vi "战舰移动限制+导弹敌机.vi"() -> ()   [LabVIEW 2018]
panel:
  in  "敌机数量":dbl
  in  "敌机速度":dbl
  out "敌机":picture
  out "按键":dbl
  out "战舰":T1
  out "激光武器1":T2
  out "激光武器 2":T2
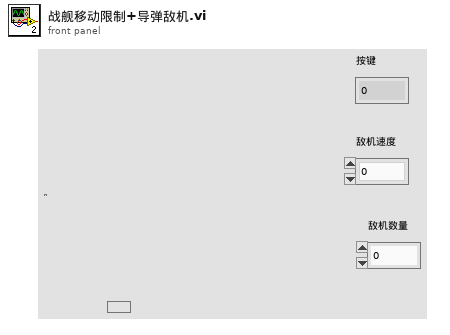
[diagram p1: front panel]
types:
  T1 = typedef "战列巡洋舰.ctl" = picture
  T2 = typedef "战列巡洋舰_激光武器.ctl" = picture
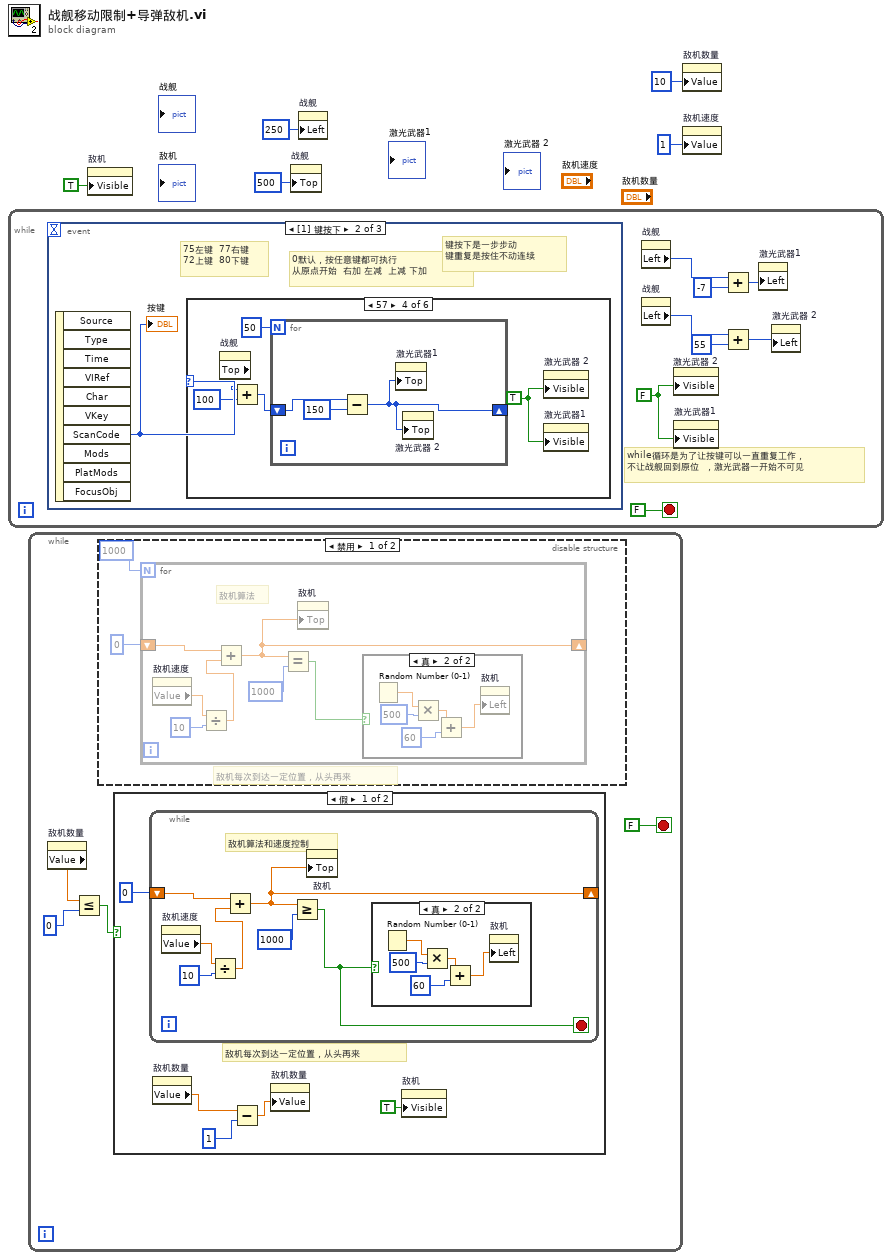
[diagram p0: block diagram]
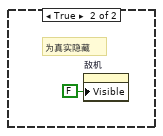
[diagram p3: hidden frame]
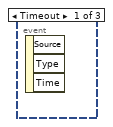
[diagram p6: hidden frame]
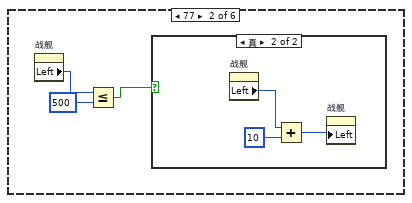
[diagram p8: hidden frame]
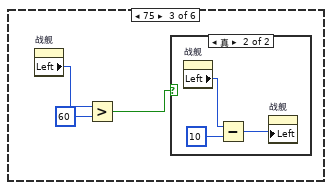
[diagram p10: hidden frame]
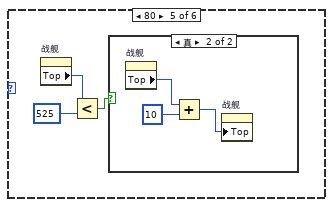
[diagram p12: hidden frame]
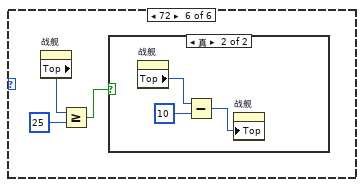
[diagram p14: hidden frame]
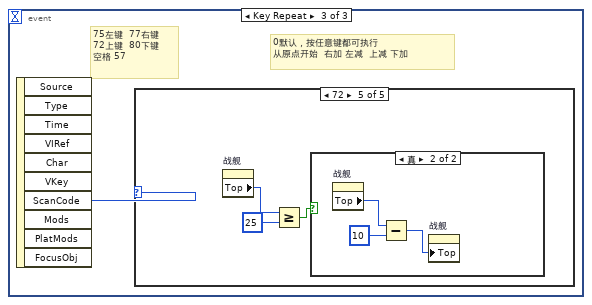
[diagram p16: hidden frame]
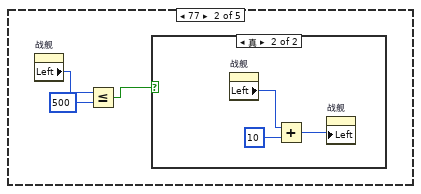
[diagram p18: hidden frame]
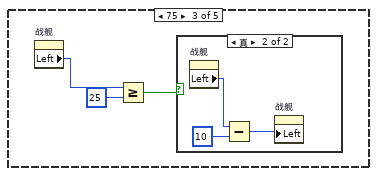
[diagram p20: hidden frame]
diagram:
  n1 = while {
    stop <- FALSE stop-if-true
    w6 = FALSE
    # "while循环是为了让按键可以一直重复工作，\n不让战舰回到原位  ，激光武器一开始不可见"
    n2 = event shown="[1] 键按下" {
      selector: _ -> [_ _ _]
      dyn-events: _ -> [_ _ _]
      timeout: _ -> [_ _ _]
      event Timeout {
        n3 = event-data() -> ()  [unwired: 1 in, 3 out]
      }
      event Key Down {
        # "键按下是一步步动\n键重复是按住不动连续"
        # "75左键  77右键\n72上键  80下键"
        # "0默认，按任意键都可执行\n从原点开始  右加 左减  上减 下加"
        n4 = event-data() -> ("ScanCode"=w14:i16)  [unwired: 1 in, 9 out]
        "按键" <- w14
        n5 = case shown="57" w14 {
          frame 0, Default {
          }
          frame 77 {
            n6 = property on="战舰" class="Pict (严格)"() -> ("Left"=w17:i32)  [unwired: 2 in, 2 out]
            n7 = Less Or Equal?(x=w17, y=500) -> (x <= y?=w15:bool)
            n8 = case shown="真" w15 {
              frame False {
              }
              frame True {
                n9 = property on="战舰" class="Pict (严格)"() -> ("Left"=w19:i32)  [unwired: 2 in, 2 out]
                n10 = Add(x=w19, y=10) -> (x+y=w20:i32)
                n11 = property on="战舰" class="Pict (严格)"("Left"=w20) -> ()  [unwired: 2 in, 2 out]
              }
            }
          }
          frame 75 {
            n12 = property on="战舰" class="Pict (严格)"() -> ("Left"=w23:i32)  [unwired: 2 in, 2 out]
            n13 = Greater?(x=w23, y=60) -> (0:w21:bool)
            n14 = case shown="真" w21 {
              frame False {
              }
              frame True {
                n15 = property on="战舰" class="Pict (严格)"() -> ("Left"=w25:i32)  [unwired: 2 in, 2 out]
                n16 = Subtract(x=w25, y=10) -> (x-y=w26:i32)
                n17 = property on="战舰" class="Pict (严格)"("Left"=w26) -> ()  [unwired: 2 in, 2 out]
              }
            }
          }
          frame 57 {
            w27 = TRUE
            n18 = property on="战舰" class="Pict (严格)"() -> ("Top"=w30:i32)  [unwired: 2 in, 2 out]
            n19 = Add(x=w30, y=100) -> (x+y=w28:i32)
            n20 = for {
              N: 50 -> [_]
              shift-right: [w32] -> _
              shift-left: w28 -> [w34]
              n21 = Subtract(x=w34, y=150) -> (x-y=w32:i32)
              n22 = property on="激光武器1" class="Pict (严格)"("Top"=w32) -> ()  [unwired: 2 in, 2 out]
              n23 = property on="激光武器 2" class="Pict (严格)"("Top"=w32) -> ()  [unwired: 2 in, 2 out]
            }
            n24 = property on="激光武器 2" class="Pict (严格)"("Visible"=w27) -> ()  [unwired: 2 in, 2 out]
            n25 = property on="激光武器1" class="Pict (严格)"("Visible"=w27) -> ()  [unwired: 2 in, 2 out]
          }
          frame 80 {
            n26 = property on="战舰" class="Pict (严格)"() -> ("Top"=w37:i32)  [unwired: 2 in, 2 out]
            n27 = Less?(x=w37, y=525) -> (x < y?=w35:bool)
            n28 = case shown="真" w35 {
              frame False {
              }
              frame True {
                n29 = property on="战舰" class="Pict (严格)"() -> ("Top"=w39:i32)  [unwired: 2 in, 2 out]
                n30 = Add(x=w39, y=10) -> (x+y=w38:i32)
                n31 = property on="战舰" class="Pict (严格)"("Top"=w38) -> ()  [unwired: 2 in, 2 out]
              }
            }
          }
          frame 72 {
            n32 = property on="战舰" class="Pict (严格)"() -> ("Top"=w43:i32)  [unwired: 2 in, 2 out]
            n33 = Greater Or Equal?(x=w43, y=25) -> (x >= y?=w42:bool)
            n34 = case shown="真" w42 {
              frame False {
              }
              frame True {
                n35 = property on="战舰" class="Pict (严格)"() -> ("Top"=w46:i32)  [unwired: 2 in, 2 out]
                n36 = Subtract(x=w46, y=10) -> (x-y=w45:i32)
                n37 = property on="战舰" class="Pict (严格)"("Top"=w45) -> ()  [unwired: 2 in, 2 out]
              }
            }
          }
        }
      }
      event Key Repeat {
        # "75左键  77右键\n72上键  80下键\n空格 57"
        # "0默认，按任意键都可执行\n从原点开始  右加 左减  上减 下加"
        n38 = event-data() -> ("ScanCode"=w47:i16)  [unwired: 1 in, 9 out]
        n39 = case shown="72" w47 {
          frame 0, Default {
          }
          frame 77 {
            n40 = property on="战舰" class="Pict (严格)"() -> ("Left"=w50:i32)  [unwired: 2 in, 2 out]
            n41 = Less Or Equal?(x=w50, y=500) -> (x <= y?=w49:bool)
            n42 = case shown="真" w49 {
              frame False {
              }
              frame True {
                n43 = property on="战舰" class="Pict (严格)"() -> ("Left"=w52:i32)  [unwired: 2 in, 2 out]
                n44 = Add(x=w52, y=10) -> (x+y=w53:i32)
                n45 = property on="战舰" class="Pict (严格)"("Left"=w53) -> ()  [unwired: 2 in, 2 out]
              }
            }
          }
          frame 75 {
            n46 = property on="战舰" class="Pict (严格)"() -> ("Left"=w56:i32)  [unwired: 2 in, 2 out]
            n47 = Greater Or Equal?(x=w56, y=25) -> (x >= y?=w55:bool)
            n48 = case shown="真" w55 {
              frame False {
              }
              frame True {
                n49 = property on="战舰" class="Pict (严格)"() -> ("Left"=w59:i32)  [unwired: 2 in, 2 out]
                n50 = Subtract(x=w59, y=10) -> (x-y=w58:i32)
                n51 = property on="战舰" class="Pict (严格)"("Left"=w58) -> ()  [unwired: 2 in, 2 out]
              }
            }
          }
          frame 80 {
            n52 = property on="战舰" class="Pict (严格)"() -> ("Top"=w62:i32)  [unwired: 2 in, 2 out]
            n53 = Less Or Equal?(x=w62, y=525) -> (x <= y?=w61:bool)
            n54 = case shown="真" w61 {
              frame False {
              }
              frame True {
                n55 = property on="战舰" class="Pict (严格)"() -> ("Top"=w64:i32)  [unwired: 2 in, 2 out]
                n56 = Add(x=w64, y=10) -> (x+y=w63:i32)
                n57 = property on="战舰" class="Pict (严格)"("Top"=w63) -> ()  [unwired: 2 in, 2 out]
              }
            }
          }
          frame 72 {
            n58 = property on="战舰" class="Pict (严格)"() -> ("Top"=w68:i32)  [unwired: 2 in, 2 out]
            n59 = Greater Or Equal?(x=w68, y=25) -> (x >= y?=w67:bool)
            n60 = case shown="真" w67 {
              frame False {
              }
              frame True {
                n61 = property on="战舰" class="Pict (严格)"() -> ("Top"=w71:i32)  [unwired: 2 in, 2 out]
                n62 = Subtract(x=w71, y=10) -> (x-y=w70:i32)
                n63 = property on="战舰" class="Pict (严格)"("Top"=w70) -> ()  [unwired: 2 in, 2 out]
              }
            }
          }
        }
      }
    }
    n64 = property on="战舰" class="Pict (严格)"() -> ("Left"=w12:i32)  [unwired: 2 in, 2 out]
    n65 = property on="战舰" class="Pict (严格)"() -> ("Left"=w8:i32)  [unwired: 2 in, 2 out]
    n66 = property on="激光武器 2" class="Pict (严格)"("Visible"=w6) -> ()  [unwired: 2 in, 2 out]
    n67 = property on="激光武器1" class="Pict (严格)"("Visible"=w6) -> ()  [unwired: 2 in, 2 out]
    n68 = Add(x=w12, y=-7) -> (x+y=w11:i32)
    n69 = Add(x=w8, y=55) -> (x+y=w7:i32)
    n70 = property on="激光武器1" class="Pict (严格)"("Left"=w11) -> ()  [unwired: 2 in, 2 out]
    n71 = property on="激光武器 2" class="Pict (严格)"("Left"=w7) -> ()  [unwired: 2 in, 2 out]
  }
  n72 = while {
    stop <- FALSE stop-if-true
    n73 = property on="敌机数量" class="DigNum (严格)"() -> ("Value"=w74:dbl)  [unwired: 2 in, 2 out]
    n74 = Less Or Equal?(x=w74, y=0) -> (x <= y?=w73:bool)
    n75 = disable-structure shown="禁用" {
      frame Disabled {
        # "敌机每次到达一定位置，从头再来"
        n76 = for {
          N: 1000 -> [_]
          shift-right: [w99] -> _
          shift-left: 0 -> [w102]
          # "敌机算法"
          n77 = property on="敌机速度" class="DigNum (严格)"() -> ("Value"=w98:dbl)  [unwired: 2 in, 2 out]
          n78 = Divide(x=w98, y=10) -> (x/y=w97:dbl)
          n79 = Add(x=w102, y=w97) -> (x+y=w99:dbl)
          n80 = Equal?(x=w99, y=1000) -> (x = y?=w100:bool)
          n81 = property on="敌机" class="Pict"("Top"=w99) -> ()  [unwired: 2 in, 2 out]
          n82 = case shown="真" w100 {
            frame False {
            }
            frame True {
              n83 = Random Number (0-1)() -> (number: 0 to 1=w107:dbl)
              n84 = Multiply(x=w107, y=500) -> (x*y=w105:dbl)
              n85 = Add(x=w105, y=60) -> (x+y=w104:dbl)
              n86 = property on="敌机" class="Pict"("Left"=w104) -> ()  [unwired: 2 in, 2 out]
            }
          }
        }
      }
      frame Enabled {
      }
    }
    n87 = case shown="假" w73 {
      frame False {
        # "敌机每次到达一定位置，从头再来"
        n88 = while {
          shift-right: [w85] -> _
          shift-left: 0 -> [w87]
          stop <- w81 stop-if-true
          # "敌机算法和速度控制"
          n89 = property on="敌机速度" class="DigNum (严格)"() -> ("Value"=w84:dbl)  [unwired: 2 in, 2 out]
          n90 = Divide(x=w84, y=10) -> (x/y=w83:dbl)
          n91 = Add(x=w87, y=w83) -> (x+y=w85:dbl)
          n92 = Greater Or Equal?(x=w85, y=1000) -> (x >= y?=w81:bool)
          n93 = property on="敌机" class="Pict"("Top"=w85) -> ()  [unwired: 2 in, 2 out]
          n94 = case shown="真" w81 {
            frame False {
            }
            frame True {
              n95 = Random Number (0-1)() -> (number: 0 to 1=w92:dbl)
              n96 = Multiply(x=w92, y=500) -> (x*y=w90:dbl)
              n97 = Add(x=w90, y=60) -> (x+y=w89:dbl)
              n98 = property on="敌机" class="Pict"("Left"=w89) -> ()  [unwired: 2 in, 2 out]
            }
          }
        }
        n99 = property on="敌机数量" class="DigNum (严格)"() -> ("Value"=w78:dbl)  [unwired: 2 in, 2 out]
        n100 = Subtract(x=w78, y=1) -> (x-y=w79:dbl)
        n101 = property on="敌机数量" class="DigNum (严格)"("Value"=w79) -> ()  [unwired: 2 in, 2 out]
        n102 = property on="敌机" class="Pict"("Visible"=TRUE ("可见")) -> ()  [unwired: 2 in, 2 out]
      }
      frame True {
        # "为真实隐藏"
        n103 = property on="敌机" class="Pict"("Visible"=FALSE ("可见")) -> ()  [unwired: 2 in, 2 out]
      }
    }
  }
  n104 = property on="敌机" class="Pict"("Visible"=TRUE ("可见")) -> ()  [unwired: 2 in, 2 out]
  n105 = property on="战舰" class="Pict (严格)"("Top"=500 ("位置:置顶")) -> ()  [unwired: 2 in, 2 out]
  n106 = property on="战舰" class="Pict (严格)"("Left"=250 ("位置:居左")) -> ()  [unwired: 2 in, 2 out]
  n107 = property on="敌机数量" class="DigNum (严格)"("Value"=10) -> ()  [unwired: 2 in, 2 out]
  n108 = property on="敌机速度" class="DigNum (严格)"("Value"=1) -> ()  [unwired: 2 in, 2 out]
